vi "Write Tag Data.vi"(8 "error in (no error)":errorcluster, 9 "Alarms Time Array":T1(array[cluster]), 11 "data":waveform(dbl)[](array[waveform])) -> (0 "error out":errorcluster, 1 "Alarm Time Array":T1(array[cluster]), 2 "DAQ value":dbl format="%0.2f", 3 "Y":dbl[](array[numeric]))   [LabVIEW 2018, in "DAQ.lvlib"]
uses:
  DAQ/DAQ.lvlib
  Tag VIs/Tag FGV Operation Enum.ctl
  <vilib>/Analysis/baseanly.llb/Mean (DBL).vi
  Shared Variables/Dynamic Shared Variables.lvlib
  <vilib>/Analysis/NI_AALBase.lvlib
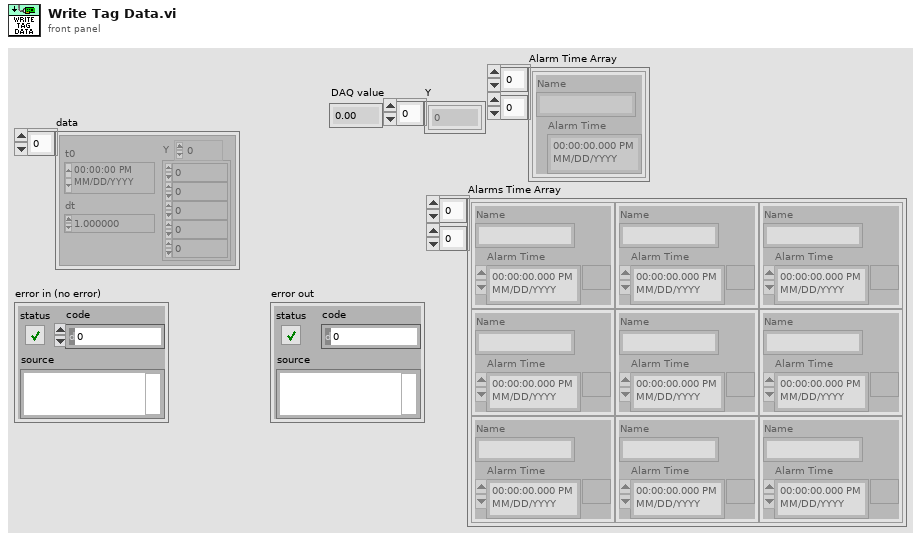
[diagram p1: front panel]
types:
  T1 = cluster{"Name":string, "Alarm Time":timestamp}[][]
  T2 = typedef "Tag FGV Operation Enum.ctl" = enum16{"Init", "Set Notification Queue", "Create Tag", "Commit", "Write Tag (Numeric)", "Write Tag (Boolean)", "Read All Tags", "Read One Tag", "Delete Tag Category", "Set Alarm Parameters (Numeric)", "Set Alarm Parameters (Boolean)", "Enable All Alarms", "Disable All Alarms", "Delete All Tags", "Read Alarms", "Ack Alarm", "Read Alarm Parameters (Numeric)", "Read Alarm Parameters (Boolean)"}
  T3 = typedef "Numeric Alarm Settings Cluster.ctl" = cluster{"enable? (F)":bool, "name":string, "alarm type":enum16{"HI_HI", "HI", "LO", "LO_LO"}, "level/change":dbl, "deadband/time":dbl, "alarm delay":dbl, "priority":u32, "ack type":enum16{"Auto", "User", "None", "Each Occurrence"}, "area":string, "description":string, "log? (T)":bool}
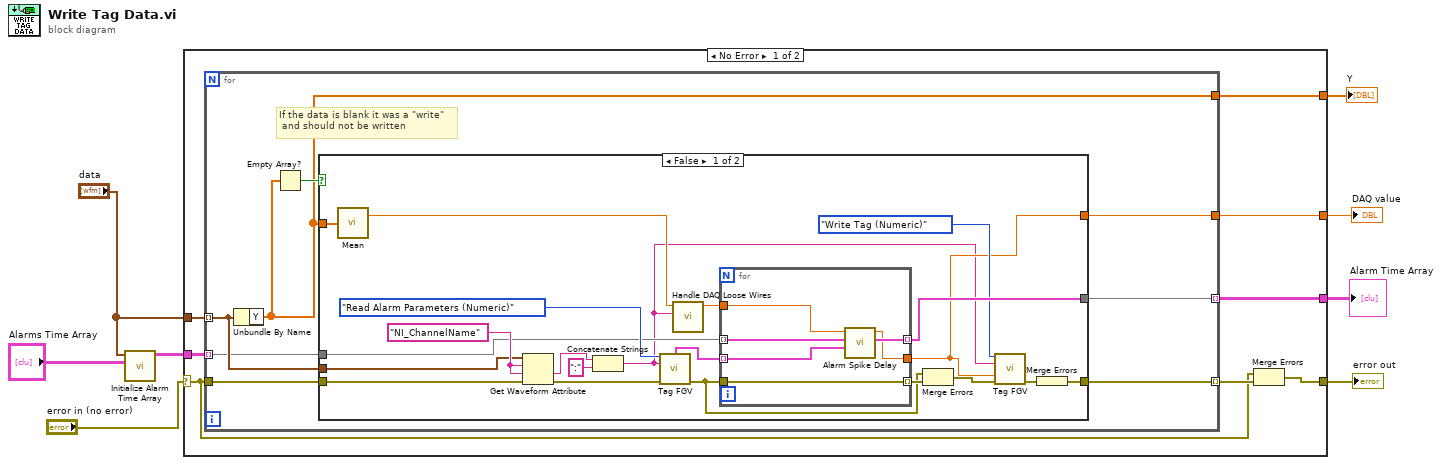
[diagram p0: block diagram]
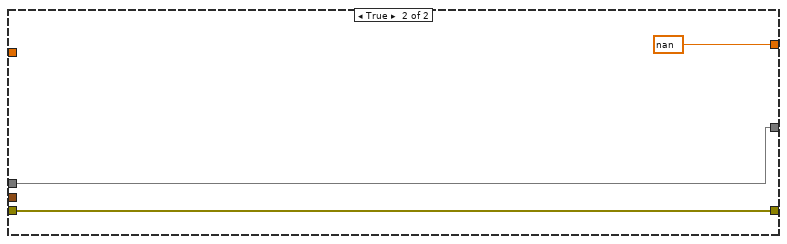
[diagram p2: hidden frame]
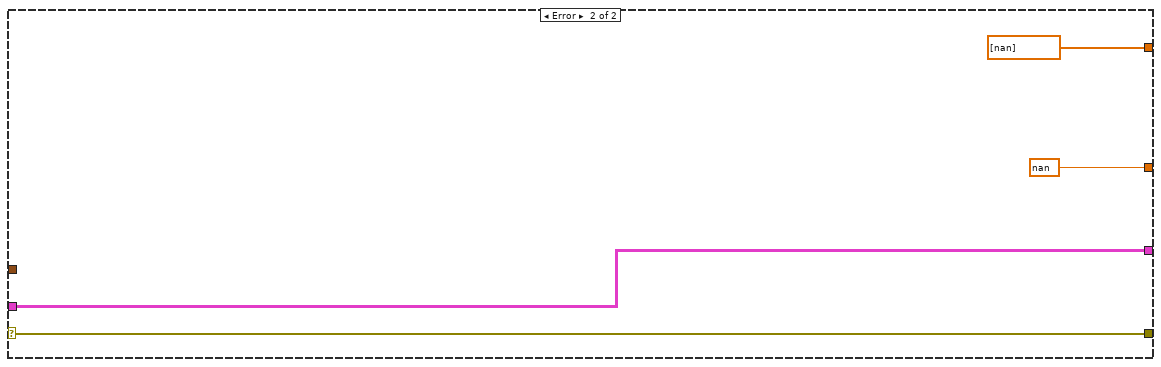
[diagram p3: hidden frame]
diagram:
  n1 = call "Initialize Alarm Time Array.vi"("Alarms Time Array in"="Alarms Time Array", "data"="data") -> ("Alarms Time Array out"=w1:T1)  [unwired: 9 in]
  n2 = case shown="No Error" "error in (no error)" {
    selector: "error in (no error)" -> [w9 w58]
    tunnel: [w10 w58] -> w8
    tunnel: "data" -> [w16 _]
    tunnel: [w15 nan ("mean")] -> w6
    tunnel: [w14 dbl[] [nan] ("Y")] -> w5
    tunnel: [w13 w55] -> w4
    tunnel: w1 -> [w12 w55]
    frame No Error {
      n3 = for {
        tunnel: w16 -> [w24] mode=indexing
        tunnel: w9 -> [w22]
        tunnel: [w21] -> w11 mode=indexing
        tunnel: [w20] -> w15
        tunnel: [w19] -> w14
        tunnel: [w18] -> w13 mode=indexing
        tunnel: w12 -> [w17] mode=indexing
        # "If the data is blank it was a \"write\"\n and should not be written"
        n4 = Unbundle By Name(w24) -> ("Y"=w19:dbl[])
        n5 = Empty Array?(array=w19) -> (empty?=w23:bool)
        n6 = case shown="False" w23 {
          tunnel: w24 -> [w44 _]
          tunnel: w19 -> [w42 _]
          tunnel: w22 -> [w43 w52]
          tunnel: [w34 w52] -> w21
          tunnel: [w29 nan ("mean")] -> w20
          tunnel: [w37 w53] -> w18
          tunnel: w17 -> [w36 w53]
          frame False {
            w45 = "NI_ChannelName" ("name")
            n7 = call-poly <vilib>:"Mean.vi"("X"=w42) -> ("mean"=w41:dbl)  [unwired: 1 out]
            n8 = Get Waveform Attribute(4:w43, 5:w45, 6:w45, 7:w44) -> (0:w35:errorcluster, 1:w27:string)  [unwired: 2 out]
            n9 = Concatenate Strings(w27, ":" ("string")) -> (w25:string)
            n10 = call "Tag FGV.vi"("Operation"=Tag_FGV_Operation_Enum."Read Alarm Parameters (Numeric)", "Tag Name"=w25, "error in (no error)"=w35) -> ("Alarm Array"=w39:T3[], "error out"=w28:errorcluster)  [unwired: 5 in, 6 out]
            n11 = call "Handle DAQ Loose Wires.vi"("Name"=w25, "Value in"=w41) -> ("Value out"=w38:dbl)  [unwired: 9 in]
            n12 = for {
              tunnel: w39 -> [w51] mode=indexing
              tunnel: w38 -> [w50]
              tunnel: [w48] -> w37 mode=indexing
              tunnel: w36 -> [w49] mode=indexing
              tunnel: [w47] -> w29
              tunnel: w28 -> [w46]
              tunnel: [w46] -> w31 mode=indexing
              n13 = call "Alarm Spike Delay.vi"("numeric alarm settings in"=w51, "Alarm Time In"=w49, "Value In"=w50) -> ("Cluster out"=w48:cluster{"Name":string, "Alarm Time":timestamp}, "Value Out"=w47:dbl)  [unwired: 7 in]
            }
            n14 = Merge Errors(w28, w31) -> (w30:errorcluster)
            n15 = call "Tag FGV.vi"("Operation"=Tag_FGV_Operation_Enum."Write Tag (Numeric)", "Tag Name"=w25, "Data"=w29, "error in (no error)"=w30) -> ("error out"=w32:errorcluster)  [unwired: 4 in, 7 out]
            n16 = Merge Errors(w32) -> (w34:errorcluster)
          }
          frame True {
          }
        }
      }
      n17 = Merge Errors(w9, w11) -> (w10:errorcluster)
    }
    frame Error {
    }
  }
  "error out" <- w8
  "DAQ value" <- w6
  "Y" <- w5
  "Alarm Time Array" <- w4
